vi "test_fileList2Tree.vi"() -> ()   [LabVIEW 2022 SP3]
uses:
  LabSSH Library/SSH Library/Connection Info..cluster.ctl
  LabSSH Library/SFTP Library/Password..cluster.ctl
  6c8e2292-66db-4772-b275-00b56b155c4b.vi
  <vilib>/Utility/error.llb/Trim Whitespace One-Sided.vi
  LabSSH Library/SFTP Library/connect_password.vi
  <vilib>/Comparison/Less/Less Functor/Less Functor.lvclass
  LabSSH Library/SFTP Library/LabSFTP.lvlib
  LabSSH Library/SSH Library/LabSSH.lvlib
panel:
  out "Array":string[](array[string])
  out "folder&file List":string
  in  "remote path":string(combo)="tvt"
  in  "user":string(combo)="tvt"
  in  "Port":u16(ring)=22 items=["22"=22, "10060"=10060, "10070"=10070, "10080"=10080, "10090"=10090]
  out "ip":string
  in  "fileTree":string(tree)
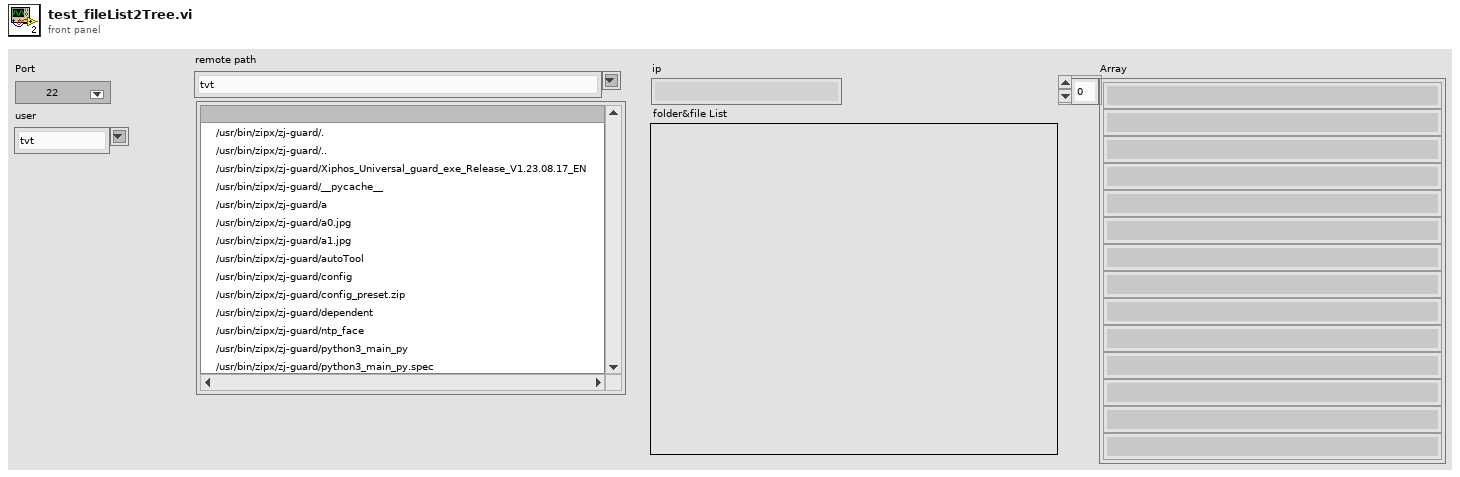
[diagram p1: front panel]
types:
  T1 = typedef "LabSFTP.lvlib/Password..cluster.ctl" = cluster{"Password":string}
  T2 = typedef "LabSSH.lvlib/Connection Info..cluster.ctl" = cluster{"Remote":string, "Username":string, "Port (22)":i32}
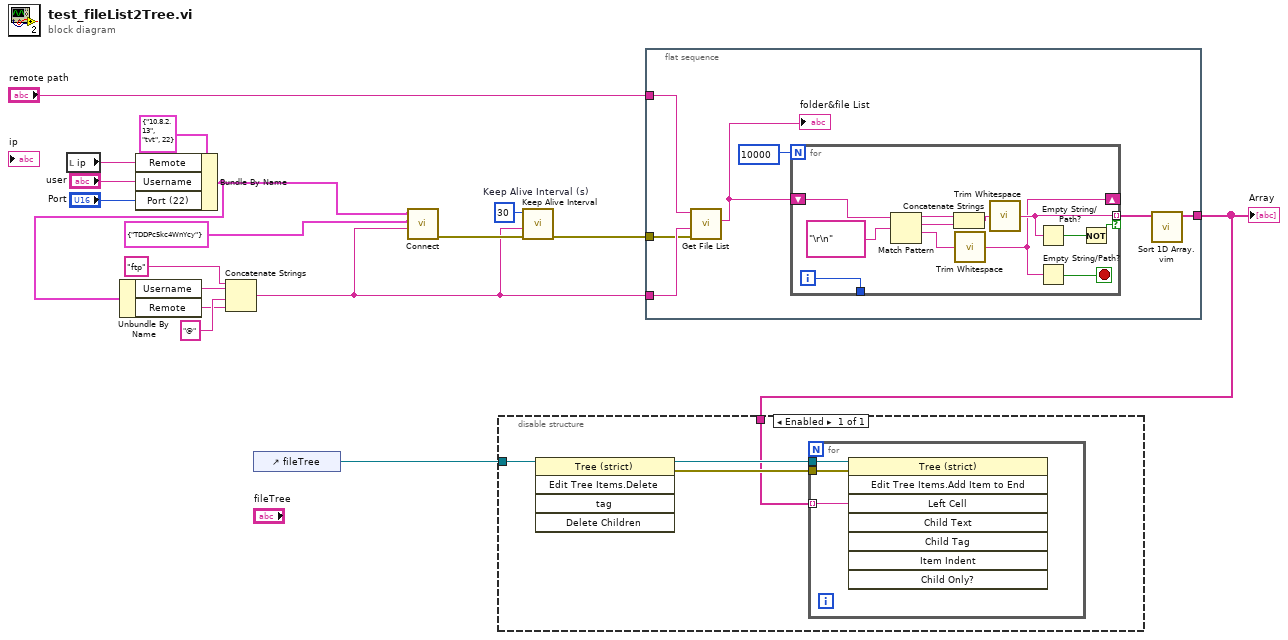
[diagram p0: block diagram]
diagram:
  w15 = 30  # Keep Alive Interval (s)
  n1 = local read "ip"() -> (w12:string)
  n2 = Bundle By Name(cluster=T2 {"Remote"="10.8.2.13", "Username"="tvt", "Port (22)"=22} ("Connection Info."), "Remote"=w12, "Username"="user", "Port (22)"="Port") -> (w5:T2)
  n3 = Unbundle By Name(w5) -> ("Username"=w7:string, "Remote"=w8:string)
  n4 = Concatenate Strings("ftp" ("string"), w7, "@" ("string"), w8) -> (w4:string)
  n5 = control-ref of="fileTree"() -> (w17:refnum<vi>)
  n6 = call-poly "Connect.vi"("Connection Name"=w4, "Password"=T1 {"Password"="TDDPc5kc4WnYcy"}, "Connection Info."=w5) -> ("error out"=w16:errorcluster)  [unwired: 6 in, 2 out]
  n7 = disable-structure shown="Enabled" {
    disable-tunnel: w17 -> [w21]
    disable-tunnel: w1 -> [w18]
    frame Enabled {
      n8 = invoke on="Invoke Node" class="Tree (strict)" method="Edit Tree Items.Delete"(reference=w21) -> (reference out=w20:refnum<vi>, error out=w19:errorcluster)  [unwired: 4 in, 3 out]
      n9 = for {
        tunnel: w20 -> [w24]
        tunnel: w19 -> [w23]
        tunnel: w18 -> [w22] mode=indexing
        n10 = invoke on="Invoke Node" class="Tree (strict)" method="Edit Tree Items.Add Item to End"(reference=w24, error in=w23, "Left Cell"=w22) -> ()  [unwired: 5 in, 8 out]
      }
    }
  }
  n11 = call "Keep Alive Interval.vi"("error in (no error)"=w16, "Connection Name"=w4, "Keep Alive Interval (s)"=w15) -> ("error out"=w3:errorcluster)  [unwired: 8 in]
  n12 = flat-sequence {
    tunnel: w4 -> [w31]
    tunnel: w3 -> [w30]
    tunnel: "remote path" -> [w26]
    tunnel: [w25] -> w1
    frame #0 {
      n13 = call "Get File List.vi"("error in (no error)"=w30, "Connection Name"=w31, "Remote Path"=w26) -> ("File List"=w28:string)  [unwired: 6 in, 2 out]
      "folder&file List" <- w28
      n14 = for {
        N: 10000 -> [_]
        tunnel: [w40] -> w27 mode=indexing if=w38
        shift-right: [w34] -> _
        shift-left: w28 -> [w43]
        tunnel: [w32] -> _
        i -> [w32]
        stop <- w33 stop-if-true
        n15 = Match Pattern(string=w43, regular expression="\r\n") -> (before substring=w41:string, match substring=w36:string, after substring=w35:string)  [unwired: 1 in, 1 out]
        n16 = Concatenate Strings(w41, w36) -> (w37:string)
        n17 = call <vilib>:"Trim Whitespace.vi"("string"=w35) -> ("trimmed string"=w34:string)  [unwired: 1 in]
        n18 = call <vilib>:"Trim Whitespace.vi"("string"=w37) -> ("trimmed string"=w40:string)  [unwired: 1 in]
        n19 = Empty String/Path?(string/path=w40) -> (empty?=w39:bool)
        n20 = Empty String/Path?(string/path=w34) -> (empty?=w33:bool)
        n21 = Not(x=w39) -> (.not. x?=w38:bool)
      }
      n22 = call "Sort 1D Array.vim"("unsorted array"=w27) -> ("sorted array"=w25:string[])  [unwired: 10 in]
    }
  }
  "Array" <- w1
